vi "单帧回看.vi"() -> ()   [LabVIEW 2018]
uses:
  <vilib>/vision/NI_Vision_Development_Module.lvlib
panel:
  out "单帧实际显示":string
  out "叠加实际显示":string
  out "单帧像素显示":string
  out "叠加像素显示":string
  out "当前可回看帧":i32
  in  "取消按钮":bool
  out "单帧火焰":T1(plugin-control)
  out "叠加火焰":T1(plugin-control)
  in  "请输入需要查看的帧数":dbl=1.0 min=1.0 max=241.0
  # "单帧回看"
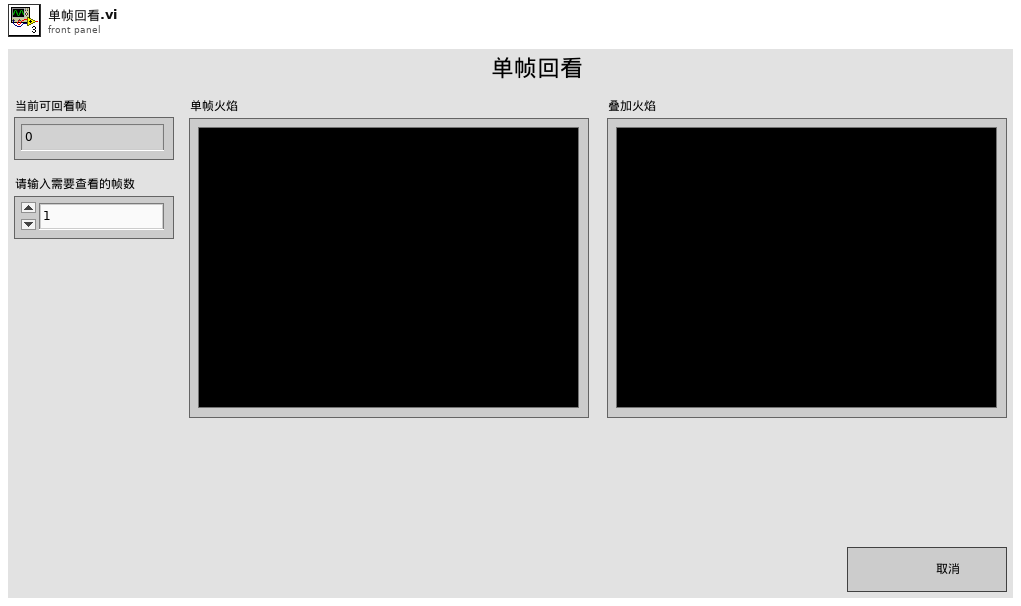
[diagram p1: front panel]
types:
  T1 = typedef "IMAQ Image.ctl" = refnum<image>
  T2 = typedef "Image Type" = u32
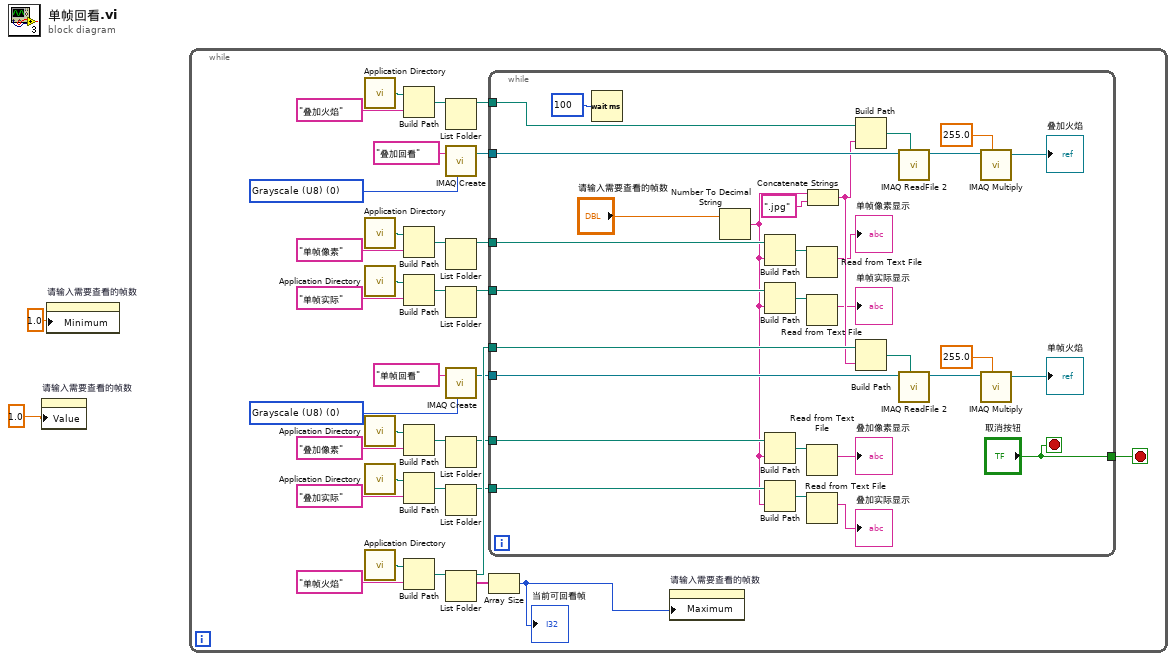
[diagram p0: block diagram]
diagram:
  n1 = property on="请输入需要查看的帧数" class="DigNum (严格)"("Value"=1.0 ("数据输入界限:最小值")) -> ()  [unwired: 2 in, 2 out]
  n2 = property on="请输入需要查看的帧数" class="DigNum (严格)"("Minimum"=1.0 ("数据输入界限:最小值")) -> ()  [unwired: 2 in, 2 out]
  n3 = while {
    stop <- w27 stop-if-true
    w25 = T2 0 items=["Grayscale (U8)", "Grayscale (I16)", "Grayscale (SGL)", "Complex (CSG)", "RGB (U32)", "HSL (U32)", "RGB (U64)", "Grayscale (U16)"] ("Image Type")
    w23 = T2 0 items=["Grayscale (U8)", "Grayscale (I16)", "Grayscale (SGL)", "Complex (CSG)", "RGB (U32)", "HSL (U32)", "RGB (U64)", "Grayscale (U16)"] ("Image Type")
    n4 = call <vilib>:"Application Directory.vi"() -> ("Application Directory"=w35:path)
    n5 = call <vilib>:"Application Directory.vi"() -> ("Application Directory"=w16:path)
    n6 = call <vilib>:"Application Directory.vi"() -> ("Application Directory"=w15:path)
    n7 = call <vilib>:"Application Directory.vi"() -> ("Application Directory"=w9:path)
    n8 = call <vilib>:"Application Directory.vi"() -> ("Application Directory"=w10:path)
    n9 = call <vilib>:"Application Directory.vi"() -> ("Application Directory"=w34:path)
    n10 = Build Path(base path=w35, name or relative path="叠加火焰" ("名称或相对路径")) -> (appended path=w30:path)
    n11 = Build Path(base path=w16, name or relative path="单帧像素" ("名称或相对路径")) -> (appended path=w18:path)
    n12 = Build Path(base path=w15, name or relative path="单帧实际" ("名称或相对路径")) -> (appended path=w13:path)
    n13 = Build Path(base path=w9, name or relative path="叠加像素" ("名称或相对路径")) -> (appended path=w7:path)
    n14 = Build Path(base path=w10, name or relative path="叠加实际" ("名称或相对路径")) -> (appended path=w12:path)
    n15 = Build Path(base path=w34, name or relative path="单帧火焰" ("名称或相对路径")) -> (appended path=w31:path)
    n16 = List Folder(path=w30) -> (path out=w28:path)  [unwired: 3 in, 3 out]
    n17 = call "IMAQ Create"("Image Name"="叠加回看", "Image Type"=w23) -> ("New Image"=w21:T1)  [unwired: 3 in, 1 out]
    n18 = List Folder(path=w18) -> (path out=w6:path)  [unwired: 3 in, 3 out]
    n19 = List Folder(path=w13) -> (path out=w5:path)  [unwired: 3 in, 3 out]
    n20 = call "IMAQ Create"("Image Name"="单帧回看", "Image Type"=w25) -> ("New Image"=w22:T1)  [unwired: 3 in, 1 out]
    n21 = List Folder(path=w7) -> (path out=w4:path)  [unwired: 3 in, 3 out]
    n22 = List Folder(path=w12) -> (path out=w3:path)  [unwired: 3 in, 3 out]
    n23 = List Folder(path=w31) -> (path out=w29:path, filenames=w20:string[])  [unwired: 3 in, 2 out]
    n24 = while {
      tunnel: w29 -> [w65]
      tunnel: w28 -> [w60]
      tunnel: w21 -> [w57]
      tunnel: w22 -> [w56]
      tunnel: ["取消按钮"] -> w27
      tunnel: w6 -> [w49]
      tunnel: w5 -> [w48]
      tunnel: w4 -> [w47]
      tunnel: w3 -> [w46]
      stop <- "取消按钮" stop-if-true
      n25 = Wait (ms)(milliseconds to wait=u32 100 ("等待时间（毫秒）")) -> ()  [unwired: 1 out]
      n26 = Number To Decimal String(number="请输入需要查看的帧数") -> (decimal integer string=w45:string)  [unwired: 1 in]
      n27 = Build Path(base path=w49, name or relative path=w45) -> (appended path=w44:path)
      n28 = Build Path(base path=w48, name or relative path=w45) -> (appended path=w42:path)
      n29 = Build Path(base path=w47, name or relative path=w45) -> (appended path=w41:path)
      n30 = Build Path(base path=w46, name or relative path=w45) -> (appended path=w40:path)
      n31 = Read from Text File(file (use dialog)=w44) -> (text=→"单帧像素显示":string)  [unwired: 3 in, 3 out]
      n32 = Read from Text File(file (use dialog)=w42) -> (text=→"单帧实际显示":string)  [unwired: 3 in, 3 out]
      n33 = Read from Text File(file (use dialog)=w41) -> (text=→"叠加像素显示":string)  [unwired: 3 in, 3 out]
      n34 = Read from Text File(file (use dialog)=w40) -> (text=→"叠加实际显示":string)  [unwired: 3 in, 3 out]
      n35 = Concatenate Strings(w45, ".jpg" ("字符串")) -> (w50:string)
      n36 = Build Path(base path=w60, name or relative path=w50) -> (appended path=w63:path)
      n37 = Build Path(base path=w65, name or relative path=w50) -> (appended path=w64:path)
      n38 = call "IMAQ ReadFile 2"("File Path"=w63, "Image"=w57) -> ("Image Out"=w53:T1)  [unwired: 5 in, 4 out]
      n39 = call "IMAQ ReadFile 2"("File Path"=w64, "Image"=w56) -> ("Image Out"=w54:T1)  [unwired: 5 in, 4 out]
      n40 = call "IMAQ Multiply"("Image Src A"=w53, "Constant"=255.0) -> ("Image Dst Out"=→"叠加火焰":T1)  [unwired: 5 in, 1 out]
      n41 = call "IMAQ Multiply"("Image Src A"=w54, "Constant"=255.0) -> ("Image Dst Out"=→"单帧火焰":T1)  [unwired: 5 in, 1 out]
    }
    n42 = Array Size(array=w20) -> (size(s)=w19:i32)
    "当前可回看帧" <- w19
    n43 = property on="请输入需要查看的帧数" class="DigNum (严格)"("Maximum"=w19) -> ()  [unwired: 2 in, 2 out]
  }
